vi "spilib_read.vi"(8 "error in (no error)":errorcluster, 10 "recv_size":i32, 11 "handle":i32) -> (0 "error out":errorcluster, 2 "recv_buf":i8[](array[numeric]), 3 "handle out":i32)   [LabVIEW 2017]
uses:
  <vilib>/Utility/error.llb/Error Cluster From Error Code.vi
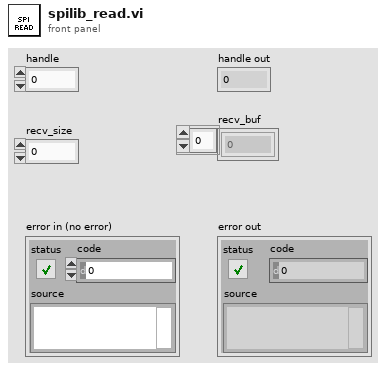
[diagram p1: front panel]
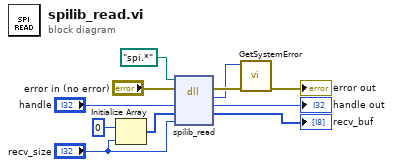
[diagram p0: block diagram]
diagram:
  n1 = Initialize Array(i8 0, "recv_size") -> (w2:i8[])
  n2 = dll-call lib="?" fn="spilib_read"(path in=path "spi.*", error in="error in (no error)", "handle"="handle", "recv_buf"=w2, "size"="recv_size") -> (error out=w10:errorcluster, "return type"=w8:i32, "handle"=→"handle out":i32, "recv_buf"=→"recv_buf":i8[])  [unwired: 2 in, 1 out]
  n3 = call <vilib>:"GetSystemError.vi"("error in (no error)"=w10, "Retval"=w8) -> ("error out"=→"error out":errorcluster)  [unwired: 9 in]
